vi "Global 5.vi"() -> ()   [LabVIEW 2018]
panel:
  out "Thermometer":dbl(slide) scale=0.0..100.0
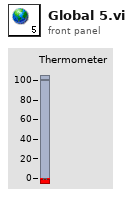
[diagram p1: front panel]
diagram:
